vi "Multiplier to color converter.vi"(4 "Multiplier":T1) -> (1 "Multiplier to color":u32(colorbox))   [LabVIEW 2018, in "Enum to Color Converter.lvlib"]
uses:
  Multiplier--control.ctl
  Enum to Color Converter.lvlib
  Resistor Band Colors/Resistor Band Colors.lvlib
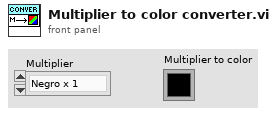
[diagram p1: front panel]
types:
  T1 = typedef "Multiplier--control.ctl" = enum16{"Negro x 1", "Marron x 10", "Rojo x 100", "Naranja x 1K", "Amarillo x 10K", "Verde x 100K", " Azul x 1M", "Violeta x 10M ", "Oro x 0.1", "Plata x 0.01"}
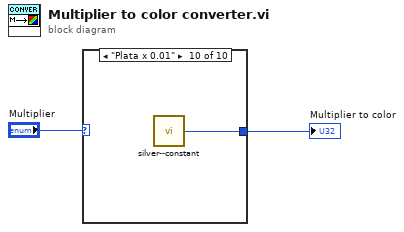
[diagram p0: block diagram]
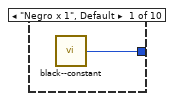
[diagram p2: hidden frame]
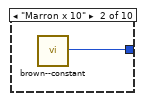
[diagram p3: hidden frame]
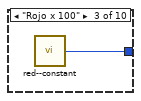
[diagram p4: hidden frame]
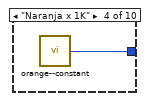
[diagram p5: hidden frame]
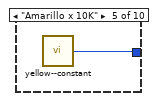
[diagram p6: hidden frame]
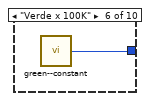
[diagram p7: hidden frame]
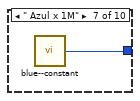
[diagram p8: hidden frame]
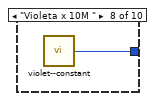
[diagram p9: hidden frame]
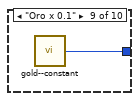
[diagram p10: hidden frame]
diagram:
  n1 = case shown="\"Plata x 0.01\"" "Multiplier" {
    tunnel: [w3 w4 w5 w6 w7 w8 w9 w10 w11 w12] -> w1
    frame "Negro x 1", Default {
      n2 = call "black--constant.vi"() -> ("Negro"=w3:u32)  [unwired: 5 in]
    }
    frame "Marron x 10" {
      n3 = call "brown--constant.vi"() -> ("brown"=w4:u32)  [unwired: 5 in]
    }
    frame "Rojo x 100" {
      n4 = call "red--constant.vi"() -> ("red"=w5:u32)  [unwired: 5 in]
    }
    frame "Naranja x 1K" {
      n5 = call "orange--constant.vi"() -> ("orange"=w6:u32)  [unwired: 5 in]
    }
    frame "Amarillo x 10K" {
      n6 = call "yellow--constant.vi"() -> ("yellow"=w7:u32)  [unwired: 5 in]
    }
    frame "Verde x 100K" {
      n7 = call "green--constant.vi"() -> ("green"=w8:u32)  [unwired: 5 in]
    }
    frame " Azul x 1M" {
      n8 = call "blue--constant.vi"() -> ("blue"=w9:u32)  [unwired: 5 in]
    }
    frame "Violeta x 10M " {
      n9 = call "violet--constant.vi"() -> ("violet"=w10:u32)  [unwired: 5 in]
    }
    frame "Oro x 0.1" {
      n10 = call "gold--constant.vi"() -> ("Gold"=w11:u32)  [unwired: 5 in]
    }
    frame "Plata x 0.01" {
      n11 = call "silver--constant.vi"() -> ("silver"=w12:u32)  [unwired: 5 in]
    }
  }
  "Multiplier to color" <- w1
